vi "Instrument Search.vi"(0 "Instrument List":T1[](array[typedef]) {"Status" format="%.0x"}, 1 "Instruments":T2[](array[typedef]), 2 "Name":string) -> (3 "VISA resource names":refnum<visa-resource-name>[](array[refnum]), 4 "Wait Times (mS)":u32[](array[numeric]), 6 "Instrument Array":T1[](array[typedef]) {"Status" format="%.0x"})   [LabVIEW 2021]
uses:
  Sub Controls/Instrument Match.ctl
  Sub Controls/Instrument IDN.ctl
  <vilib>/regexp/Match Regular Expression.xnode
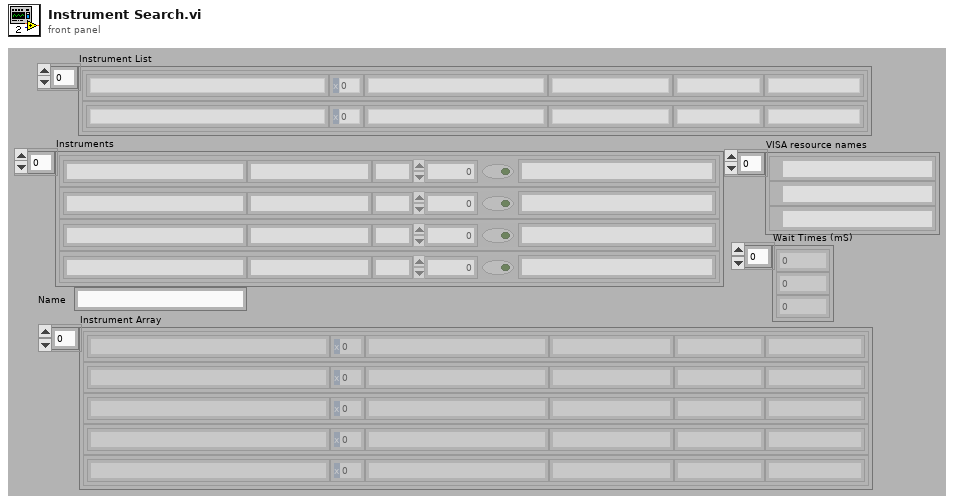
[diagram p1: front panel]
types:
  T1 = typedef "Instrument IDN.ctl" = cluster{"VISA Address":string, "Status":u16, "Manufacturer":string, "Model":string, "Info":string, "Info 2":string, "Misc Data":variant}
  T2 = typedef "Instrument Match.ctl" = cluster{"Model":string, "Manufacturer":string, "Term Character":string, "Wait Time (mS)":u32, "Wait for SRQ":bool, "Type":string}
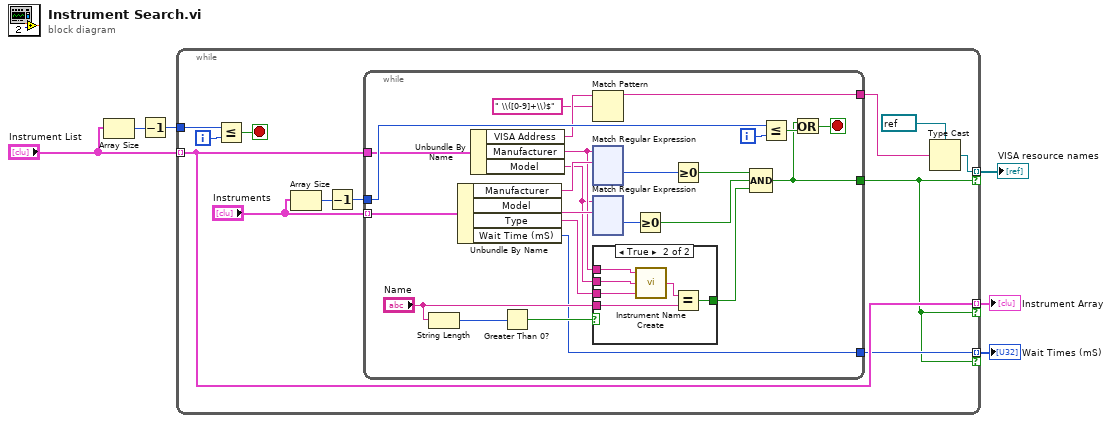
[diagram p0: block diagram]
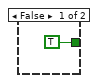
[diagram p2: hidden frame]
diagram:
  n1 = Array Size(array="Instrument List") -> (size(s)=w5:i32)
  n2 = Decrement(x=w5) -> (x-1=w4:i32)
  n3 = while {
    tunnel: "Instrument List" -> [w9] mode=indexing
    tunnel: w4 -> [w17]
    tunnel: [w10] -> w3 mode=indexing if=w7
    tunnel: [w9] -> w2 mode=indexing if=w7
    tunnel: [w8] -> w1 mode=indexing if=w7
    i -> [w18]
    stop <- w12 stop-if-true
    n4 = Less Or Equal?(x=w17, y=w18) -> (x <= y?=w12:bool)
    n5 = Array Size(array="Instruments") -> (size(s)=w16:i32)
    n6 = Decrement(x=w16) -> (x-1=w14:i32)
    n7 = while {
      tunnel: "Instruments" -> [w42] mode=indexing
      tunnel: w9 -> [w36]
      tunnel: w14 -> [w40]
      tunnel: [w37] -> w7
      tunnel: [w33] -> w13
      tunnel: [w19] -> w8
      i -> [w38]
      stop <- w41 stop-if-true
      n8 = String Length(string="Name") -> (length=w29:i32)
      n9 = Unbundle By Name(w42) -> ("Manufacturer"=w25:string, "Model"=w26:string, "Type"=w27:string, "Wait Time (mS)"=w19:u32)
      n10 = Unbundle By Name(w36) -> ("VISA Address"=w32:string, "Manufacturer"=w23:string, "Model"=w22:string)
      n11 = Greater Than 0?(x=w29) -> (x > 0?=w24:bool)
      n12 = Match Pattern(string=w32, regular expression=" \\([0-9]+\\)$") -> (before substring=w33:string)  [unwired: 1 in, 3 out]
      n13 = xnode "Match Regular Expression"("input string"=w23, "regular expression"=w25) -> ("offset past match"=w21:i32)  [unwired: 4 in, 4 out]
      n14 = xnode "Match Regular Expression"("input string"=w22, "regular expression"=w26) -> ("offset past match"=w20:i32)  [unwired: 4 in, 4 out]
      n15 = case shown="True" w24 {
        tunnel: "Name" -> [_ w283]
        tunnel: [TRUE ("T") w282] -> w28
        tunnel: w27 -> [_ w280]
        tunnel: w22 -> [_ w279]
        tunnel: w23 -> [_ w278]
        frame False {
        }
        frame True {
          n16 = call "Instrument Name Create.vi"("Instrument Type"=w280, "Model"=w279, "Manufacturer"=w278) -> ("Name"=w281:string)
          n17 = Equal?(x=w281, y=w283) -> (x = y?=w282:bool)
        }
      }
      n18 = Greater Or Equal To 0?(x=w20) -> (x >= 0?=w34:bool)
      n19 = Greater Or Equal To 0?(x=w21) -> (x >= 0?=w35:bool)
      n20 = Compound Arithmetic op=AND(w35, w34, w28) -> (w37:bool)
      n21 = Less Or Equal?(x=w40, y=w38) -> (x <= y?=w39:bool)
      n22 = Or(x=w37, y=w39) -> (x .or. y?=w41:bool)
    }
    n23 = Type Cast(type=refnum<visa-resource-name> refnum ("VISA resource name"), x=w13) -> (*(type *) &x=w10:refnum<visa-resource-name>)
  }
  "VISA resource names" <- w3
  "Instrument Array" <- w2
  "Wait Times (mS)" <- w1
